vi "loadAODOwfparamsfromsettingsfile.vi"(0 "sertting":string) -> ()   [LabVIEW 2015]
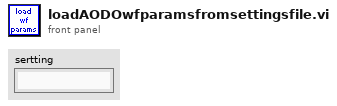
[diagram p1: front panel]
types:
  T1 = cluster{"settings names":string[], "settings locations":path[]}
  T2 = cluster{"AO parameters":cluster{"AOtab":dbl, "Repeats":dbl, "Cycles":dbl, "Start amplitude (V)":dbl, "Baseline (V)":dbl, "Step size (V)":dbl, "DC (%)":dbl, "Sampling frequency (Hz)":dbl, "Period (ms)":dbl, "Offset (V)":dbl, "Amplitude (V)":dbl, "Frequency":dbl, "Tri Repeats":dbl, "phase shift (ms)":dbl, "Pulses":dbl, "Matlab wave file":path, "Tri phase":dbl, "padding value":dbl}[], "DO parameters":cluster{"Digital DC (%)":dbl, "Digital phase":dbl, "Digital Freq (Hz)":dbl, "Sampling frequency (Hz)":dbl, "Digital time offset (s) ":dbl, "padding value":dbl, "matlab wave file":path, "DOtab":dbl}[]}
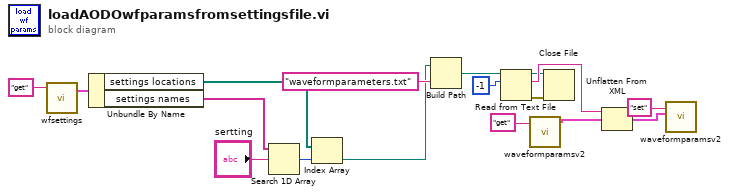
[diagram p0: block diagram]
diagram:
  n1 = call "wfsettings.vi"("command"="get") -> ("wfsettings out"=w15:T1)  [unwired: 2 in, 1 out]
  n2 = Unbundle By Name(w15) -> ("settings locations"=w13:path[], "settings names"=w14:string[])
  n3 = Search 1D Array(1D array=w14, element="sertting") -> (index of element=w17:i32)  [unwired: 1 in]
  n4 = Index Array(array=w13, index=w17) -> (element=w5:path)
  n5 = Build Path(base path=w5, name or relative path="waveformparameters.txt") -> (appended path=w7:path)
  n6 = Read from Text File(file (use dialog)=w7, count=-1) -> (refnum out=w10:refnum<file>, text=w12:string, error out=w11:errorcluster)  [unwired: 2 in, 1 out]
  n7 = call "waveformparamsv2.vi"("command"="get") -> ("Params out"=w3:T2)  [unwired: 4 in, 2 out]
  n8 = Close File(refnum=w10, error in=w11) -> ()  [unwired: 2 out]
  n9 = Unflatten From XML(xml string=w12, type=w3) -> (value=w1:T2)  [unwired: 1 in, 1 out]
  n10 = call "waveformparamsv2.vi"("command"="set", "Params in"=w1) -> ()  [unwired: 3 in, 3 out]
